vi "Check If Pixels Belong In Sector.vi"() -> (3 "FIFO Timeout?":bool)   [LabVIEW 2013]
uses:
  Single Sector Pixel Cluster.ctl
  Globals/Sector Parameter Global.vi
  Globals/Pixel Location Global.vi
  <vilib>/rvi/FIFO/Fifo_Resource/nirvififoEmulationReadFpgaImpl.vi
  <vilib>/rvi/DataTransferAndStorage/Container/Common/niFpgaContainerGetUniqueNameForEmu.vi
  <vilib>/rvi/FIFO/Fifo_Resource/nirvififoEmulationWriteFpgaImpl.vi
  <vilib>/rvi/DataTransferAndStorage/Container/XNode/niFpgaContainer.xnode
  <vilib>/rvi/FIFO/Fifo_Resource/nirvififoEmulationRead.vi
  <vilib>/rvi/FIFO/Fifo_Resource/nirvififoEmulationWrite.vi
panel:
  out "End of  Data?":bool
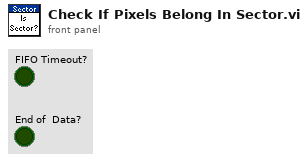
[diagram p1: front panel]
types:
  T1 = typedef "Single Sector Pixel Cluster.ctl" = cluster{"Sector #":u8, "Pixel Value":u8}
  T2 = typedef "Sector Parameter Cluster.ctl" = cluster{"Start Angle":fxp<+/-,17,2>, "End Angle":fxp<+/-,17,2>, "Inner Radius":u16, "Outter Radius":u16, "Hinge X":u16, "Hinge Y":u16, "NumWingSectors":u8}
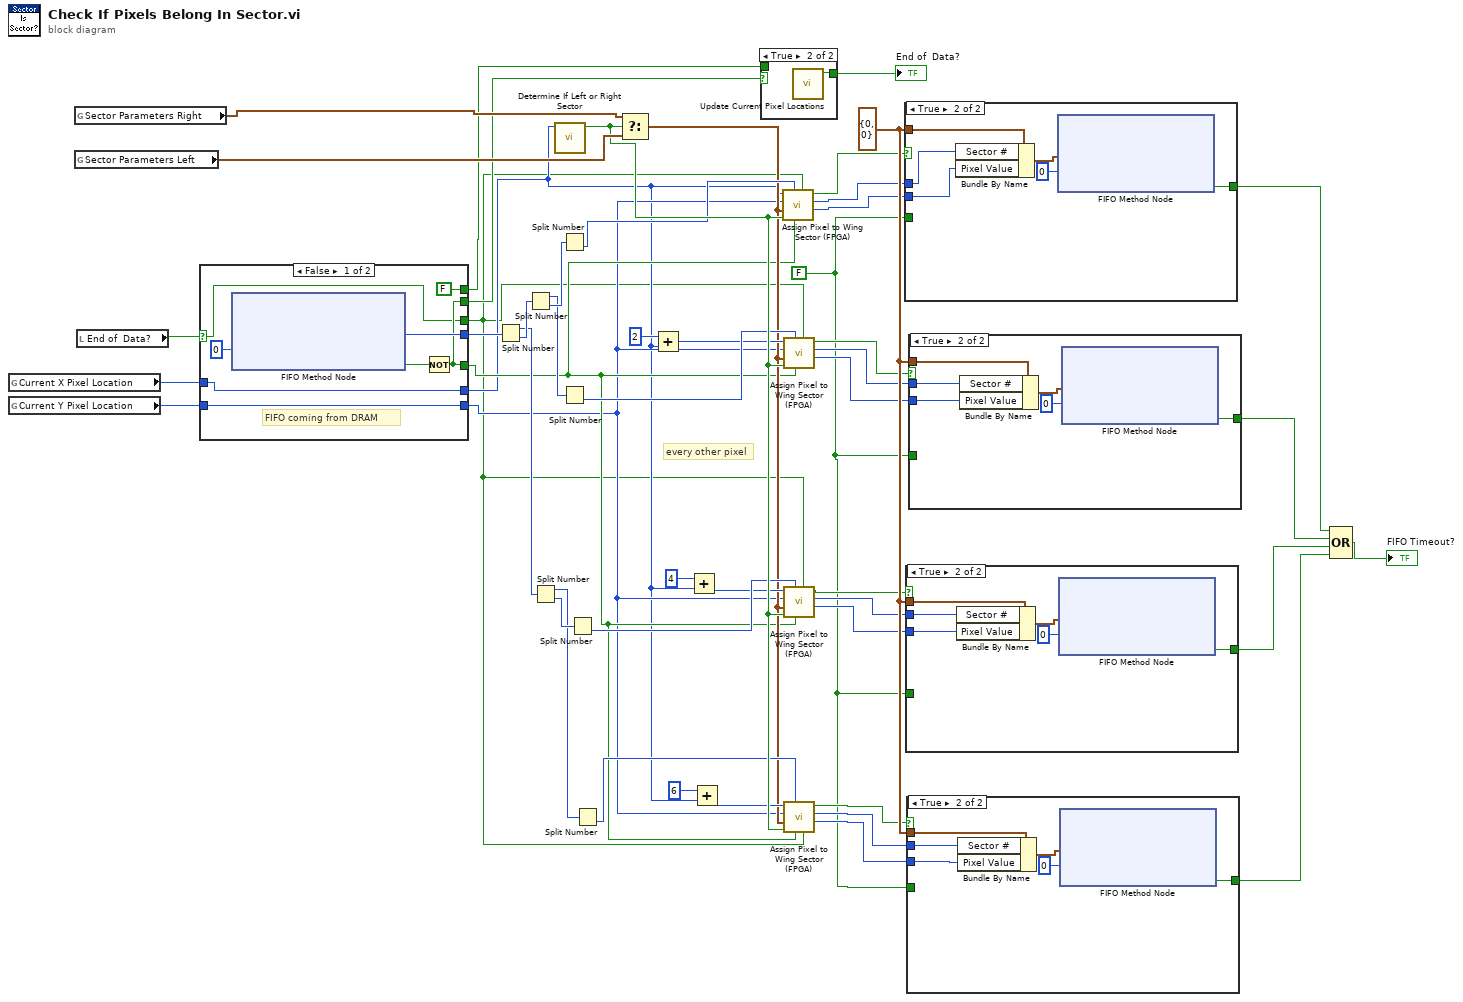
[diagram p0: block diagram]
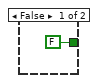
[diagram p3: hidden frame]
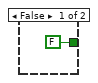
[diagram p4: hidden frame]
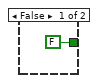
[diagram p5: hidden frame]
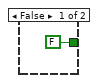
[diagram p6: hidden frame]
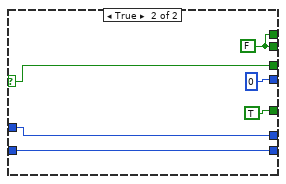
[diagram p7: hidden frame]
diagram:
  w28 = FALSE
  w41 = T1 {"Sector #"=0, "Pixel Value"=0} ("Single Sector Pixel")
  # "every other pixel"
  n1 = global read "Pixel Location Global.vi" "Current X Pixel Location"() -> (w2:u16)
  n2 = global read "Pixel Location Global.vi" "Current Y Pixel Location"() -> (w4:u16)
  n3 = global read "Sector Parameter Global.vi" "Sector Parameters Right"() -> (w48:T2)
  n4 = global read "Sector Parameter Global.vi" "Sector Parameters Left"() -> (w47:T2)
  n5 = local read "End of  Data?"() -> (w6:bool)
  n6 = case shown="False" w6 {
    selector: w6 -> [w51 w59]
    tunnel: [w55 TRUE ("Timed Out?")] -> w9
    tunnel: [w57 u64 0 ("Element")] -> w46
    tunnel: [w55 w62] -> w8
    tunnel: [FALSE ("Timed Out?") w62] -> w7
    tunnel: [w53 w60] -> w5
    tunnel: w4 -> [w53 w60]
    tunnel: [w52 w61] -> w3
    tunnel: w2 -> [w52 w61]
    tunnel: [w51 w59] -> w1
    frame False {
      # "FIFO coming from DRAM"
      n7 = xnode ("FIFO Method Node")("Timeout"=0) -> ("Element"=w57:u64, "Timed Out?"=w56:bool)  [unwired: 1 in, 1 out]
      n8 = Not(x=w56) -> (.not. x?=w55:bool)
    }
    frame True {
      w62 = FALSE ("Timed Out?")
    }
  }
  n9 = Split Number(x=w46) -> (hi(x)=w26:u32, lo(x)=w27:u32)
  n10 = Split Number(x=w27) -> (hi(x)=w24:u16, lo(x)=w25:u16)
  n11 = Split Number(x=w26) -> (hi(x)=w22:u16, lo(x)=w23:u16)
  n12 = call "Determine If Left or Right Sector.vi"("X Pixel Location"=w3) -> ("Right Sector?"=w21:bool)  [unwired: 10 in]
  n13 = Split Number(x=w25) -> (lo(x)=w20:u8)  [unwired: 1 out]
  n14 = Split Number(x=w24) -> (lo(x)=w19:u8)  [unwired: 1 out]
  n15 = Split Number(x=w23) -> (lo(x)=w18:u8)  [unwired: 1 out]
  n16 = Split Number(x=w22) -> (lo(x)=w17:u8)  [unwired: 1 out]
  n17 = Select(t=w48, s=w21, f=w47) -> (s? t:f=w10:T2)
  n18 = Add(x=u16 2, y=w3) -> (x+y=w13:u16)
  n19 = Add(x=u16 4, y=w3) -> (x+y=w12:u16)
  n20 = Add(x=u16 6, y=w3) -> (x+y=w11:u16)
  n21 = case shown="True" w8 {
    tunnel: [w65 w66] -> w50
    tunnel: w7 -> [w65 _]
    frame False {
    }
    frame True {
      n22 = call "Update Current Pixel Locations.vi"() -> ("End of data?"=w66:bool)  [unwired: 11 in]
    }
  }
  "End of  Data?" <- w50
  n23 = call "Assign Pixel to Wing Sector (FPGA).vi"("End of Data?"=w1, "Valid Data?"=w9, "Pixel Intensity In"=w20, "Right Wing?"=w21, "Sector Parameters"=w10, "Pixel Y"=w5, "Pixel X"=w3) -> ("Pixel Intensity Out"=w38:u8, "sector #"=w39:u8, "output valid"=w40:bool)  [unwired: 2 in]
  n24 = call "Assign Pixel to Wing Sector (FPGA).vi"("End of Data?"=w1, "Valid Data?"=w9, "Pixel Intensity In"=w19, "Right Wing?"=w21, "Sector Parameters"=w10, "Pixel Y"=w5, "Pixel X"=w13) -> ("Pixel Intensity Out"=w35:u8, "sector #"=w36:u8, "output valid"=w37:bool)  [unwired: 2 in]
  n25 = call "Assign Pixel to Wing Sector (FPGA).vi"("End of Data?"=w1, "Valid Data?"=w9, "Pixel Intensity In"=w18, "Right Wing?"=w21, "Sector Parameters"=w10, "Pixel Y"=w5, "Pixel X"=w12) -> ("Pixel Intensity Out"=w32:u8, "sector #"=w33:u8, "output valid"=w34:bool)  [unwired: 2 in]
  n26 = call "Assign Pixel to Wing Sector (FPGA).vi"("End of Data?"=w1, "Valid Data?"=w9, "Pixel Intensity In"=w17, "Right Wing?"=w21, "Sector Parameters"=w10, "Pixel Y"=w5, "Pixel X"=w11) -> ("Pixel Intensity Out"=w29:u8, "sector #"=w30:u8, "output valid"=w31:bool)  [unwired: 2 in]
  n27 = case shown="True" w40 {
    tunnel: w41 -> [_ w70]
    tunnel: [FALSE ("Timed Out?") w71] -> w45
    tunnel: w39 -> [_ w69]
    tunnel: w38 -> [_ w68]
    tunnel: w28 -> [_ _]
    frame False {
    }
    frame True {
      n28 = Bundle By Name(cluster=w70, "Sector #"=w69, "Pixel Value"=w68) -> (w72:T1)
      n29 = xnode ("FIFO Method Node")("Element"=w72, "Timeout"=0) -> ("Timed Out?"=w71:bool)  [unwired: 1 in, 1 out]
    }
  }
  n30 = case shown="True" w34 {
    tunnel: w41 -> [_ w80]
    tunnel: [FALSE ("Timed Out?") w77] -> w43
    tunnel: w33 -> [_ w75]
    tunnel: w32 -> [_ w76]
    tunnel: w28 -> [_ _]
    frame False {
    }
    frame True {
      n31 = Bundle By Name(cluster=w80, "Sector #"=w75, "Pixel Value"=w76) -> (w78:T1)
      n32 = xnode ("FIFO Method Node")("Element"=w78, "Timeout"=0) -> ("Timed Out?"=w77:bool)  [unwired: 1 in, 1 out]
    }
  }
  n33 = case shown="True" w31 {
    tunnel: w41 -> [_ w87]
    tunnel: [FALSE ("Timed Out?") w84] -> w42
    tunnel: w30 -> [_ w82]
    tunnel: w29 -> [_ w83]
    tunnel: w28 -> [_ _]
    frame False {
    }
    frame True {
      n34 = Bundle By Name(cluster=w87, "Sector #"=w82, "Pixel Value"=w83) -> (w85:T1)
      n35 = xnode ("FIFO Method Node")("Element"=w85, "Timeout"=0) -> ("Timed Out?"=w84:bool)  [unwired: 1 in, 1 out]
    }
  }
  n36 = case shown="True" w37 {
    tunnel: w41 -> [_ w94]
    tunnel: [FALSE ("Timed Out?") w91] -> w44
    tunnel: w36 -> [_ w89]
    tunnel: w35 -> [_ w90]
    tunnel: w28 -> [_ _]
    frame False {
    }
    frame True {
      n37 = Bundle By Name(cluster=w94, "Sector #"=w89, "Pixel Value"=w90) -> (w92:T1)
      n38 = xnode ("FIFO Method Node")("Element"=w92, "Timeout"=0) -> ("Timed Out?"=w91:bool)  [unwired: 1 in, 1 out]
    }
  }
  n39 = Compound Arithmetic op=OR(w45, w44, w43, w42) -> (→"FIFO Timeout?":bool)
